vi "close.vi"(8 "error in (no error)":errorcluster, 11 "niDAQmxAO in":refnum<class "niDAQmxAO.lvclass">) -> (0 "error out":errorcluster)   [LabVIEW 2011, in "Hardware.lvlib" / "Channels.lvlib" / "niDAQmxAO.lvclass"]
uses:
  niDAQmxAO.lvclass
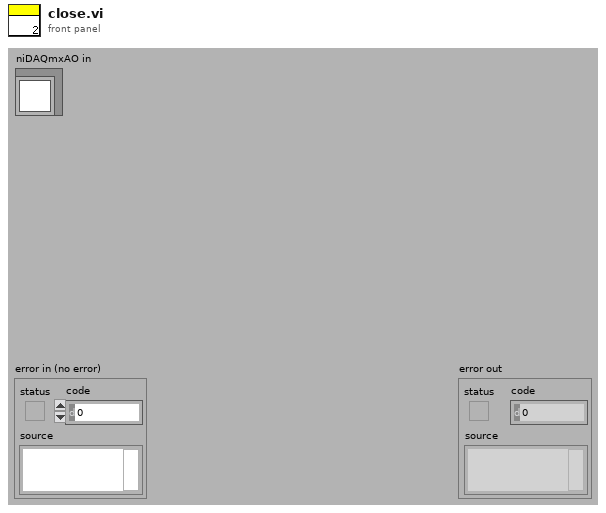
[diagram p1: front panel]
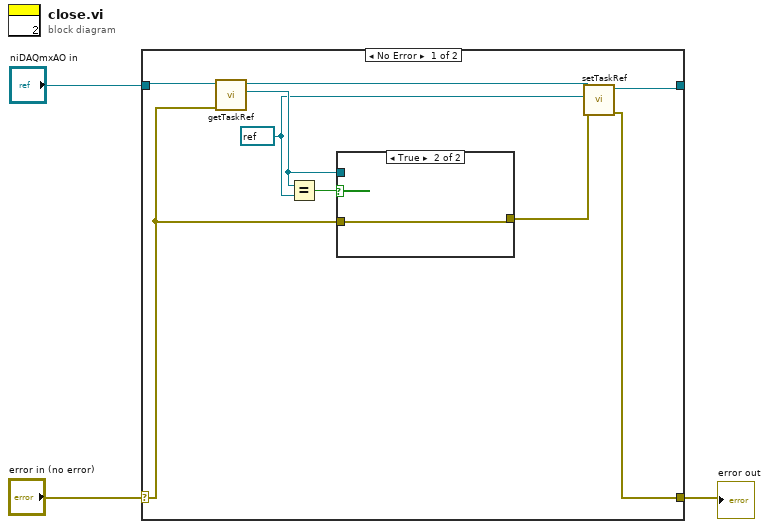
[diagram p0: block diagram]
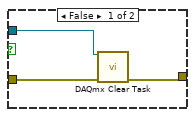
[diagram p2: hidden frame]
diagram:
  n1 = case shown="No Error" "error in (no error)" {
    selector: "error in (no error)" -> [w7 w17]
    tunnel: "niDAQmxAO in" -> [w10 w18]
    tunnel: [w11 w18] -> _
    tunnel: [w4 w17] -> w1
    frame No Error {
      w6 = refnum<k21> refnum ("DAQmx Task Ref")
      n2 = call "getTaskRef.vi"("error in (no error)"=w7, "niDAQmxAO.lvclass in"=w10) -> ("DAQmx Task Ref"=w8:refnum<k21>, "niDAQmxAO.lvclass out"=w12:refnum<class "niDAQmxAO.lvclass">)  [unwired: 7 in, 1 out]
      n3 = Equal?(x=w8, y=w6) -> (x = y?=w9:bool)
      n4 = case shown="True" w9 {
        tunnel: w8 -> [w15 _]
        tunnel: w7 -> [w14 w16]
        tunnel: [w13 w16] -> w5
        frame False {
          n5 = call <vilib>:"DAQmx Clear Task.vi"("task in"=w15, "error in"=w14) -> ("error out"=w13:errorcluster)  [unwired: 13 in]
        }
        frame True {
        }
      }
      n6 = call "setTaskRef.vi"("error in (no error)"=w5, "DAQmx Task Ref"=w6, "niDAQmxAO.lvclass in"=w12) -> ("error out"=w4:errorcluster, "niDAQmxAO.lvclass out"=w11:refnum<class "niDAQmxAO.lvclass">)  [unwired: 7 in]
    }
    frame Error {
    }
  }
  "error out" <- w1
